vi "ResultSORTER.vi"(2 "Array 4":string[](array[string]), 3 "Array 3":dbl[][](array[numeric]) format="%.2f") -> (0 "Array":T1[](array[typedef]) {"F2-Value overall" format="%.2f"; "tauerror" format="%.2f"; "Lifetime[ns]" format="%.2f"; "F2-Value TAC" format="%.2f"})   [LabVIEW 2009]
uses:
  spotproperties.ctl
panel:
  out "SpotProperties":T1 {"F2-Value overall" format="%.2f"; "tauerror" format="%.2f"; "Lifetime[ns]" format="%.2f"; "F2-Value TAC" format="%.2f"}
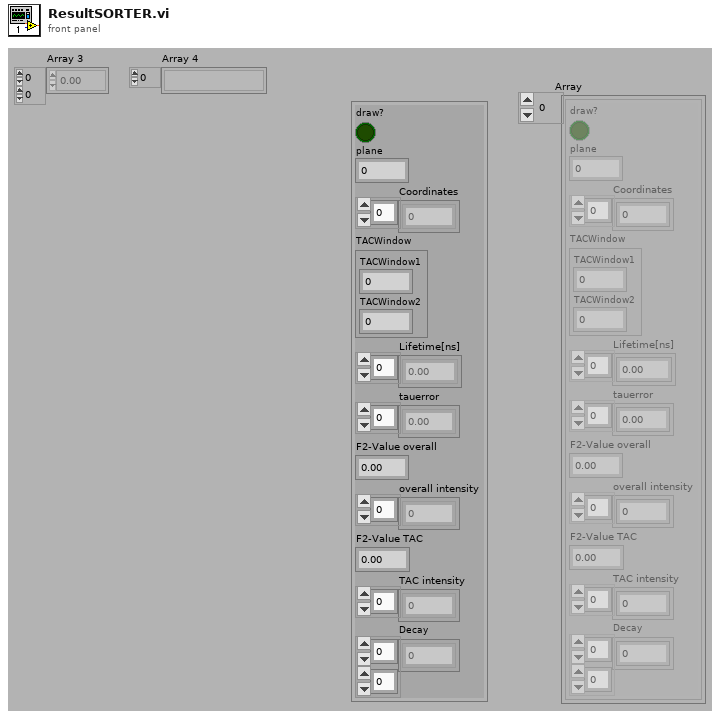
[diagram p1: front panel]
types:
  T1 = typedef "spotproperties.ctl" = cluster{"draw?":bool, "plane":u32, "Coordinates":i32[], "TACWindow":cluster{"TACWindow1":i32, "TACWindow2":i32}, "Lifetime[ns]":ext[], "tauerror":dbl[], "F2-Value overall":dbl, "overall intensity":u32[], "F2-Value TAC":dbl, "TAC intensity":u32[], "Decay":u32[][]}
  T2 = cluster{"draw?":bool, "plane":u32, "Coordinates":i32[], "TACWindow":cluster{"TACWindow1":i32, "TACWindow2":i32}, "Lifetime[ns]":ext[], "tauerror":dbl[], "F2-Value overall":dbl, "overall intensity":u32[], "F2-Value TAC":dbl, "TAC intensity":u32[], "Decay":u32[][]}
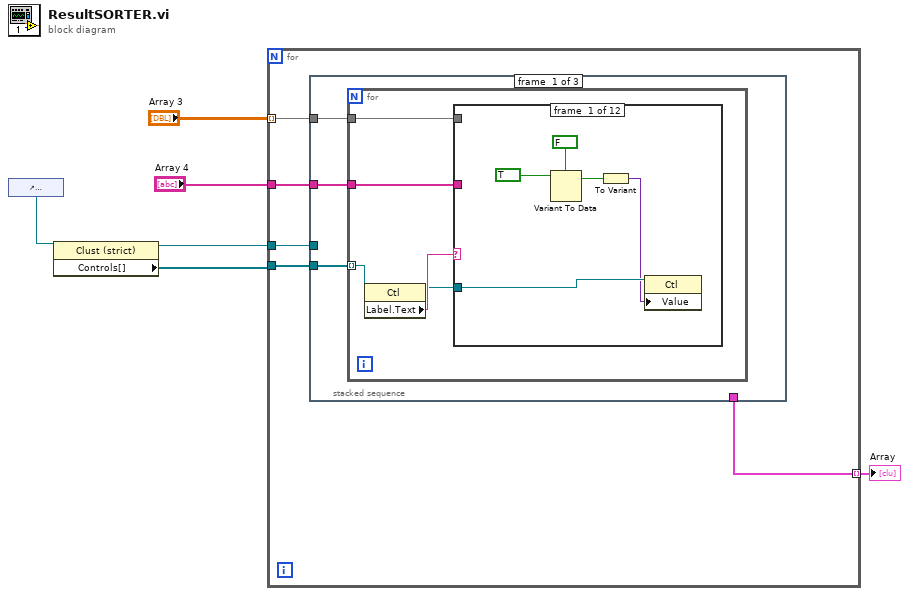
[diagram p0: block diagram]
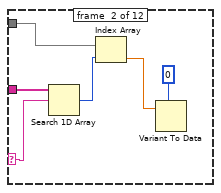
[diagram p2: hidden frame]
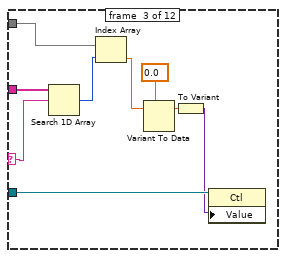
[diagram p3: hidden frame]
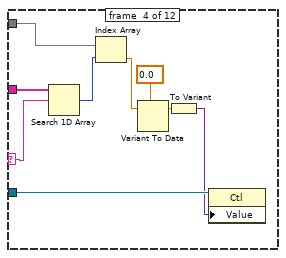
[diagram p4: hidden frame]
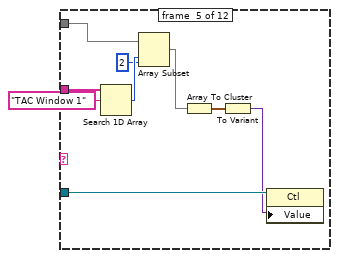
[diagram p5: hidden frame]
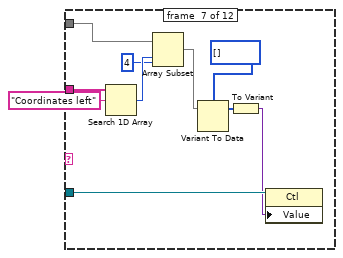
[diagram p7: hidden frame]
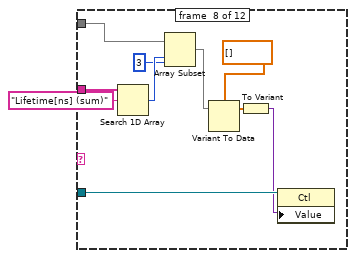
[diagram p8: hidden frame]
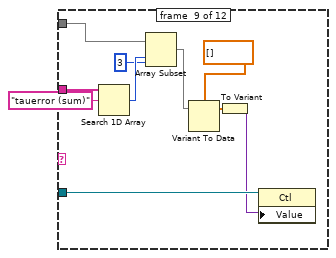
[diagram p9: hidden frame]
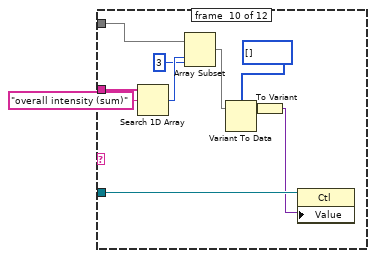
[diagram p10: hidden frame]
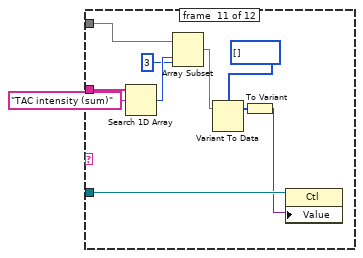
[diagram p11: hidden frame]
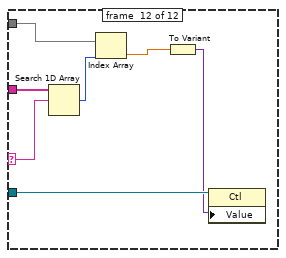
[diagram p12: hidden frame]
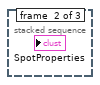
[diagram p13: hidden frame]
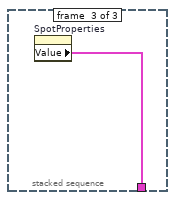
[diagram p14: hidden frame]
diagram:
  n1 = control-ref of="SpotProperties"() -> (w2:refnum<vi>)
  n2 = property class="Clust (strict)"(reference=w2) -> (reference out=w6:refnum<vi>, "Controls[]"=w5:refnum<vi>[])  [unwired: 1 in, 1 out]
  n3 = for {
    tunnel: "Array 3" -> [w10] mode=indexing
    tunnel: w5 -> [w11]
    tunnel: "Array 4" -> [w9]
    tunnel: w6 -> [w8]
    tunnel: [w7] -> w1 mode=indexing
    n4 = stacked-sequence {
      tunnel: w11 -> [w14 _ _]
      tunnel: w10 -> [w13 _ _]
      tunnel: [_ _ w115] -> w7
      tunnel: w9 -> [w12 _ _]
      tunnel: w8 -> [_ _ _]
      frame #0 {
        n5 = for {
          tunnel: w14 -> [w19] mode=indexing
          tunnel: w13 -> [w17]
          tunnel: w12 -> [w16]
          n6 = property class="Ctl"(reference=w19) -> (reference out=w15:refnum<vi>, "Label.Text"=w18:string)  [unwired: 1 in, 1 out]
          n7 = case shown="\"plane\"" w18 {
            selector: w18 -> [_ w28 w37 w46 _ _ _ _ _ _ _ w110]
            tunnel: w17 -> [_ w30 w39 w48 w57 _ w67 w77 w87 w97 w107 w114]
            tunnel: w16 -> [_ w29 w38 w47 w56 _ w66 w76 w86 w96 w106 w113]
            tunnel: w15 -> [w22 _ w35 w44 w54 _ w64 w74 w84 w94 w104 w111]
            frame #0 {
              n8 = Variant To Data(Variant=TRUE, type=FALSE) -> (data=w21:bool)  [unwired: 1 in, 1 out]
              n9 = To Variant(anything=w21) -> (Variant=w20:variant)
              n10 = property class="Ctl"(reference=w22, "Value"=w20) -> ()  [unwired: 1 in, 2 out]
            }
            frame #1 {
              n11 = Search 1D Array(1D array=w29, element=w28) -> (index of element=w27:i32)  [unwired: 1 in]
              n12 = Index Array(array=w30, index=w27) -> (element=w26:dbl)
              n13 = Variant To Data(Variant=w26, type=u16 0) -> ()  [unwired: 1 in, 2 out]
            }
            frame #2 {
              n14 = Search 1D Array(1D array=w38, element=w37) -> (index of element=w36:i32)  [unwired: 1 in]
              n15 = Index Array(array=w39, index=w36) -> (element=w34:dbl)
              n16 = Variant To Data(Variant=w34, type=0.0) -> (data=w33:dbl)  [unwired: 1 in, 1 out]
              n17 = To Variant(anything=w33) -> (Variant=w31:variant)
              n18 = property class="Ctl"(reference=w35, "Value"=w31) -> ()  [unwired: 1 in, 2 out]
            }
            frame #3 {
              n19 = Search 1D Array(1D array=w47, element=w46) -> (index of element=w45:i32)  [unwired: 1 in]
              n20 = Index Array(array=w48, index=w45) -> (element=w43:dbl)
              n21 = Variant To Data(Variant=w43, type=0.0) -> (data=w42:dbl)  [unwired: 1 in, 1 out]
              n22 = To Variant(anything=w42) -> (Variant=w40:variant)
              n23 = property class="Ctl"(reference=w44, "Value"=w40) -> ()  [unwired: 1 in, 2 out]
            }
            frame #4 {
              n24 = Search 1D Array(1D array=w56, element="TAC Window 1") -> (index of element=w55:i32)  [unwired: 1 in]
              n25 = Array Subset(array=w57, index=w55, length=2) -> (w50:dbl[])
              n26 = Array To Cluster(array=w50) -> (cluster=w49:cluster{"[0]":dbl, "[1]":dbl})
              n27 = To Variant(anything=w49) -> (Variant=w51:variant)
              n28 = property class="Ctl"(reference=w54, "Value"=w51) -> ()  [unwired: 1 in, 2 out]
            }
            frame #5 {
            }
            frame #6 {
              n29 = Search 1D Array(1D array=w66, element="Coordinates left") -> (index of element=w65:i32)  [unwired: 1 in]
              n30 = Array Subset(array=w67, index=w65, length=4) -> (w63:dbl[])
              n31 = Variant To Data(Variant=w63, type=u16[] [] ("Coordinates")) -> (data=w62:u16[])  [unwired: 1 in, 1 out]
              n32 = To Variant(anything=w62) -> (Variant=w58:variant)
              n33 = property class="Ctl"(reference=w64, "Value"=w58) -> ()  [unwired: 1 in, 2 out]
            }
            frame #7 {
              n34 = Search 1D Array(1D array=w76, element="Lifetime[ns] (sum)") -> (index of element=w75:i32)  [unwired: 1 in]
              n35 = Array Subset(array=w77, index=w75, length=3) -> (w73:dbl[])
              n36 = Variant To Data(Variant=w73, type=dbl[] [] ("Coordinates")) -> (data=w72:dbl[])  [unwired: 1 in, 1 out]
              n37 = To Variant(anything=w72) -> (Variant=w68:variant)
              n38 = property class="Ctl"(reference=w74, "Value"=w68) -> ()  [unwired: 1 in, 2 out]
            }
            frame #8 {
              n39 = Search 1D Array(1D array=w86, element="tauerror (sum)") -> (index of element=w85:i32)  [unwired: 1 in]
              n40 = Array Subset(array=w87, index=w85, length=3) -> (w83:dbl[])
              n41 = Variant To Data(Variant=w83, type=dbl[] [] ("Coordinates")) -> (data=w82:dbl[])  [unwired: 1 in, 1 out]
              n42 = To Variant(anything=w82) -> (Variant=w78:variant)
              n43 = property class="Ctl"(reference=w84, "Value"=w78) -> ()  [unwired: 1 in, 2 out]
            }
            frame #9 {
              n44 = Search 1D Array(1D array=w96, element="overall intensity (sum)") -> (index of element=w95:i32)  [unwired: 1 in]
              n45 = Array Subset(array=w97, index=w95, length=3) -> (w93:dbl[])
              n46 = Variant To Data(Variant=w93, type=u16[] [] ("Coordinates")) -> (data=w92:u16[])  [unwired: 1 in, 1 out]
              n47 = To Variant(anything=w92) -> (Variant=w88:variant)
              n48 = property class="Ctl"(reference=w94, "Value"=w88) -> ()  [unwired: 1 in, 2 out]
            }
            frame #10 {
              n49 = Search 1D Array(1D array=w106, element="TAC intensity (sum)") -> (index of element=w105:i32)  [unwired: 1 in]
              n50 = Array Subset(array=w107, index=w105, length=3) -> (w103:dbl[])
              n51 = Variant To Data(Variant=w103, type=u16[] [] ("Coordinates")) -> (data=w102:u16[])  [unwired: 1 in, 1 out]
              n52 = To Variant(anything=w102) -> (Variant=w98:variant)
              n53 = property class="Ctl"(reference=w104, "Value"=w98) -> ()  [unwired: 1 in, 2 out]
            }
            frame #11 {
              n54 = Search 1D Array(1D array=w113, element=w110) -> (index of element=w112:i32)  [unwired: 1 in]
              n55 = Index Array(array=w114, index=w112) -> (element=w108:dbl)
              n56 = To Variant(anything=w108) -> (Variant=w109:variant)
              n57 = property class="Ctl"(reference=w111, "Value"=w109) -> ()  [unwired: 1 in, 2 out]
            }
          }
        }
      }
      frame #1 {
      }
      frame #2 {
        n58 = property on="SpotProperties" class="Cluster (strict)"() -> ("Value"=w115:T2)  [unwired: 2 in, 2 out]
      }
    }
  }
  "Array" <- w1
